vi "init asynch process.vi"(8 "error in (no error)":errorcluster, 10 "data allocations":T1, 11 "Modbus Module runtime in":refnum<class "Modbus Module runtime.lvclass">) -> (0 "error out":errorcluster, 3 "Modbus Module runtime out":refnum<class "Modbus Module runtime.lvclass">)   [LabVIEW 2014, in "Modbus Module runtime.lvclass"]
uses:
  Modbus Module runtime.lvclass
  <vilib>/NI/Tag Bus Module Framework/channel/data tables.ctl
  <vilib>/NI/Tag Bus/dictionary/data dictionary.lvclass
  <vilib>/NI/Tag Bus/dictionary table pair.ctl
  <vilib>/NI/Tag Bus/table/data table.ctl
  message to background process.ctl
  command enum.ctl
  asynch process references.ctl
  response from background process.ctl
  response enum.ctl
  Modbus Module runtime.lvclass/Modbus Module runtime.ctl
  modbus asynch.vi
  <vilib>/NI/Tag Bus/table/data table.lvlib
  <vilib>/NI/Tag Bus/tag bus.lvlib
  <vilib>/NI/Tag Bus Module Framework/channel/TBM channel.lvclass
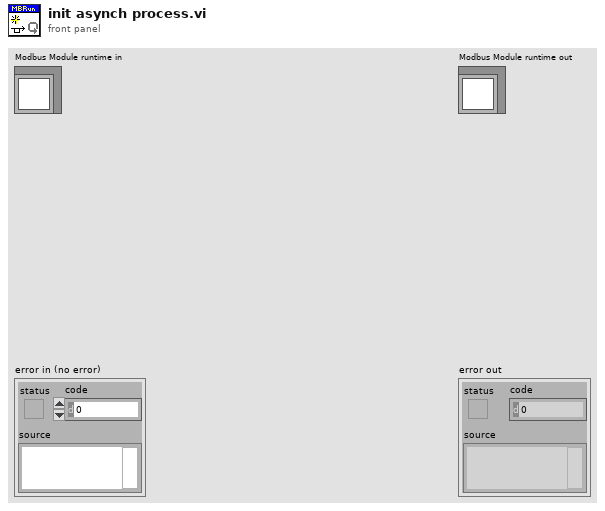
[diagram p1: front panel]
types:
  T1 = typedef "TBM channel.lvclass/data tables.ctl" = cluster{"input data":T2, "processing parameter":T2, "processing result":T2, "output data":T2}
  T2 = typedef "tag bus.lvlib/dictionary table pair.ctl" = cluster{"data dictionary":refnum<class "data dictionary.lvclass">, "data table":T3}
  T3 = typedef "tag bus.lvlib/data table.lvlib/data table.ctl" = cluster{"Double":dbl[], "Single":sgl[], "I64":i64[], "I32":i32[], "I16":i16[], "I8":i8[], "U64":u64[], "U32":u32[], "U16":u16[], "U8":u8[], "Boolean":bool[], "String":string[], "Array of Double":cluster{"DBL Array":dbl[]}[], "Array of Single":cluster{"SGL Array":sgl[]}[], "Array of I64":cluster{"I64 Array":i64[]}[], "Array of I32":cluster{"I32 Array":i32[]}[], "Array of I16":cluster{"I16 Array":i16[]}[], "Array of I8":cluster{"I8 Array":i8[]}[], "Array of U64":cluster{"U64 Array":u64[]}[], "Array of U32":cluster{"U32 Array":u32[]}[], "Array of U16":cluster{"U16 Array":u16[]}[], "Array of U8":cluster{"U8 Array":u8[]}[], "Array of Boolean":cluster{"Boolean Array":bool[]}[], "Array of String":cluster{"String Array":string[]}[]}
  T4 = typedef "Modbus Module runtime.lvclass/command enum.ctl" = enum16{"stop", "input", "output"}
  T5 = cluster{"read mode":enum16{"polling", "blocking"}, "write mode":enum16{"polling", "blocking"}}
  T6 = typedef "Modbus Module runtime.lvclass/asynch process references.ctl" = cluster{"commands":refnum<k33>, "input buffer":refnum<k33>, "output buffer":refnum<k33>, "asynch VI ref":variant, "original DVRs":refnum<data-value>[]}
  T7 = typedef "Modbus Module runtime.lvclass/response from background process.ctl" = cluster{"response enum":T8, "datapack":refnum<data-value>, "error code":i32}
  T8 = typedef "Modbus Module runtime.lvclass/response enum.ctl" = enum16{"exit", "return buffer", "error"}
  T9 = typedef "Modbus Module runtime.lvclass/message to background process.ctl" = cluster{"command enum":T4, "datapack":refnum<data-value>}
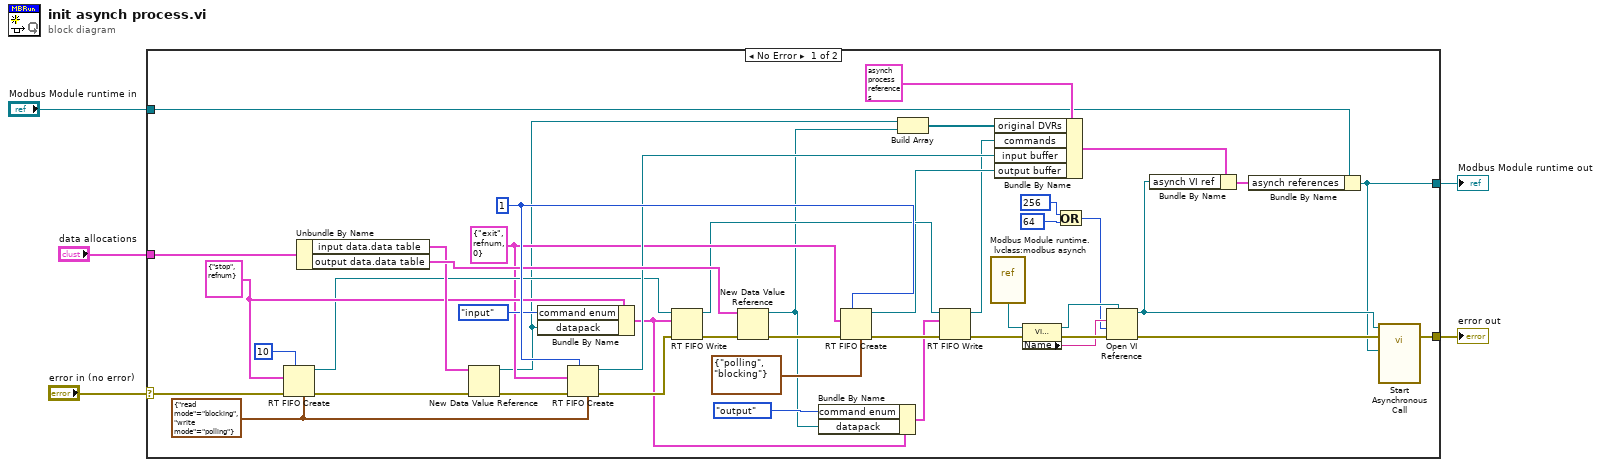
[diagram p0: block diagram]
diagram:
  n1 = case shown="No Error" "error in (no error)" {
    selector: "error in (no error)" -> [w44 w51]
    tunnel: [w35 w51] -> w4
    tunnel: [w20 w50] -> w2
    tunnel: "Modbus Module runtime in" -> [w32 w50]
    tunnel: "data allocations" -> [w31 _]
    frame No Error {
      w15 = T7 {"response enum"=enum."exit", "datapack"=refnum, "error code"=0} ("message")
      w46 = T5 {"read mode"=enum."blocking", "write mode"=enum."polling"} ("r/w modes (polling,polling)")
      w45 = u32 1 ("size (10)")
      w18 = T9 {"command enum"=enum."stop", "datapack"=refnum} ("message")
      n2 = RT FIFO Create(1:w18, 3:w44, 4:u32 10 ("size (10)"), 7:w46) -> (8:w16:refnum<k33>, 11:w23:errorcluster)  [unwired: 4 in, 1 out]
      n3 = Unbundle By Name(w31) -> ("input data.data table"=w22:T3, "output data.data table"=w28:T3)
      n4 = New Data Value Reference(data value=w22, error in=w23) -> (data value reference=w7:refnum<data-value>, error out=w29:errorcluster)
      n5 = Bundle By Name(cluster=w18, "command enum"=command_enum."input", "datapack"=w7) -> (w11:T9)
      n6 = RT FIFO Create(1:w15, 3:w29, 4:w45, 7:w46) -> (8:w19:refnum<k33>, 11:w30:errorcluster)  [unwired: 4 in, 1 out]
      n7 = RT FIFO Write(0:w16, 1:w11, 3:w30) -> (8:w14:refnum<k33>, 11:w25:errorcluster)  [unwired: 2 in, 2 out]
      n8 = New Data Value Reference(data value=w28, error in=w25) -> (data value reference=w8:refnum<data-value>, error out=w24:errorcluster)
      n9 = Bundle By Name(cluster=w11, "command enum"=command_enum."output", "datapack"=w8) -> (w9:T9)
      n10 = RT FIFO Create(1:w15, 3:w24, 4:w45, 7:T5 {"read mode"=enum."polling", "write mode"=enum."blocking"} ("r/w modes (polling,polling)")) -> (8:w13:refnum<k33>, 11:w27:errorcluster)  [unwired: 4 in, 1 out]
      n11 = Build Array(w7, w8) -> (w6:refnum<data-value>[])
      n12 = RT FIFO Write(0:w14, 1:w9, 3:w27) -> (8:w12:refnum<k33>, 11:w26:errorcluster)  [unwired: 2 in, 2 out]
      n13 = vi-ref "Modbus Module runtime.lvclass:modbus asynch.vi"() -> (w43:refnum<vi>)
      n14 = Bundle By Name(cluster=T6 {"commands"=refnum, "input buffer"=refnum, "output buffer"=refnum, "asynch VI ref"=variant, "original DVRs"=[]} ("asynch references"), "original DVRs"=w6, "commands"=w12, "input buffer"=w19, "output buffer"=w13) -> (w33:T6)
      n15 = property class="VI (strict)"(reference=w43, error in=w26) -> (reference out=w41:refnum<vi>, error out=w42:errorcluster, "Name"=w40:string)
      n16 = Or(x=256, y=64) -> (x .or. y?=w37:i32)
      n17 = Open VI Reference(type specifier VI Refnum (for type only)=w41, vi path=w40, options=w37, error in (no error)=w42) -> (vi reference=w21:refnum<vi>, error out=w36:errorcluster)  [unwired: 2 in]
      n18 = Bundle By Name(cluster=w33, "asynch VI ref"=w21) -> (w34:T6)
      n19 = Bundle By Name(cluster=w32, "asynch references"=w34) -> (w20:refnum<class "Modbus Module runtime.lvclass">)
      n20 = call-by-ref "Start Asynchronous Call"(reference=w21, error in=w36, "Modbus Module runtime in"=w20) -> (error out=w35:errorcluster)  [unwired: 10 in, 2 out]
    }
    frame Error {
    }
  }
  "error out" <- w4
  "Modbus Module runtime out" <- w2
